vi "TSI Bench Single Socket CPV Sweeps E4990A Ver3.0.vi"() -> ()   [LabVIEW 2017]
uses:
  <vilib>/Utility/file.llb/Read Delimited Spreadsheet (DBL).vi
  Test Equipment/E364x/Agilent E364X Series/Agilent E364X Series.lvlib
  Test Equipment/KE2000/Keithley 2000/Keithley 2000.lvlib
panel:
  out "Cycles":string="2000"
  in  "Tab Control":enum32{"Control"}(tab)
  in  "Measure CMin \n& CMax Only?":bool
  in  "T- CAP(fF)":dbl[](array[numeric])=[100.0, 2968.75]
  out "Diff DCAP":dbl[](array[numeric])=[0.0, 158.76451612903202, 128.65967741935475, 83.51039999999999, 79.098, 80.17639999999999, 81.14560000000002, 79.77199999999999, 91.06439999999998, 80.7144, 80.3784, 79.76879999999998, 80.59799999999998, 91.3732, 90.2772]
  out "IDD ON (uA)":string
  out "I_Stdby (uA)":string
  out "CMax(fF)":dbl
  in  "Cycle?":bool=TRUE
  out "Cycles  No":i32=2000
  out "CMin (fF)":dbl=255.30700000000002
  in  "TP":string="TSI Bench Single Socket CPV Sweep E4990A Ver3.0"
  out "Error Out":errorcluster={"status"=FALSE, "code"=1073676407, "source"="VISA Open in Agilent E364X Series.lvlib:Initialize.vi->WS1021 Screen Parts Bench Test Ver1.4.vi"}
  in  "Base Path":path=path "C:/TSI Material"
  out "Status":string="Save Data..."
  in  "Tab Control 2":T1(tab)=enum."Input Info"
  in  "AGE364X":refnum<visa-resource-name>="GPIB0::6::INSTR"
  in  "VDD/VIO":dbl[](array[numeric])=[3.3, 1.8]
  in  "I_Limit (mA)":dbl=20.0 format="%.2p"
  in  "Select CPV":i32(ring)=17 items=["CP 24V", "CP 26V", "CP 28V", "CP 30V", "CP 31V", "CP 32V", "CP 33V", "CP 34V", "CP 35V", "CP 36V", "CP 37V", "CP 38V", "CP 39V", "CP 40V", "CP 41V", "CP 42V", "CP 43V", "CP 44V", "CP 45V", "CP 46V", "CP 47V", "CP 48V", "CP 49V", "CP 50V", "CP 51V", "CP 52V", "CP 53V", "CP 54V", "CP 56V", "CP 58V", "CP 60V", "CP 62V"]
  in  "Settings":bool
  in  "Comport Setting":refnum<visa-resource-name>="COM8"
  in  "Manual Write":string
  in  "Send":bool
  in  "No of Cycles":i32=2000
  in  "AG4990A":refnum<visa-resource-name>="GPIB0::17::INSTR"
  in  "KE2000":refnum<visa-resource-name>="GPIB0::9::INSTR"
  in  "Process Stop Button":bool
  in  "Stop":bool
  in  "Error In":errorcluster
  in  "CP CYC":bool
  in  "VDD":bool
  in  "Capacitance":bool
  in  "Info":T2={"Lot"="3127C", "Wafer"="11", "Package"="BC_C", "Device"="1"}
  out "IDD":cluster{dbl[], dbl[]}(graph)
  out "Cap Plot":cluster{dbl[], dbl[]}(graph)
  # "WiSpry Inc 20 Fairbanks \nSte 198 Irvine CA 92618\n\n\n\n\nRev Date = 07/27/2021\nTP:  TSI Bench Single Socket CPV Sweep E4990A Ver3.0\nLabVIEW 2017"
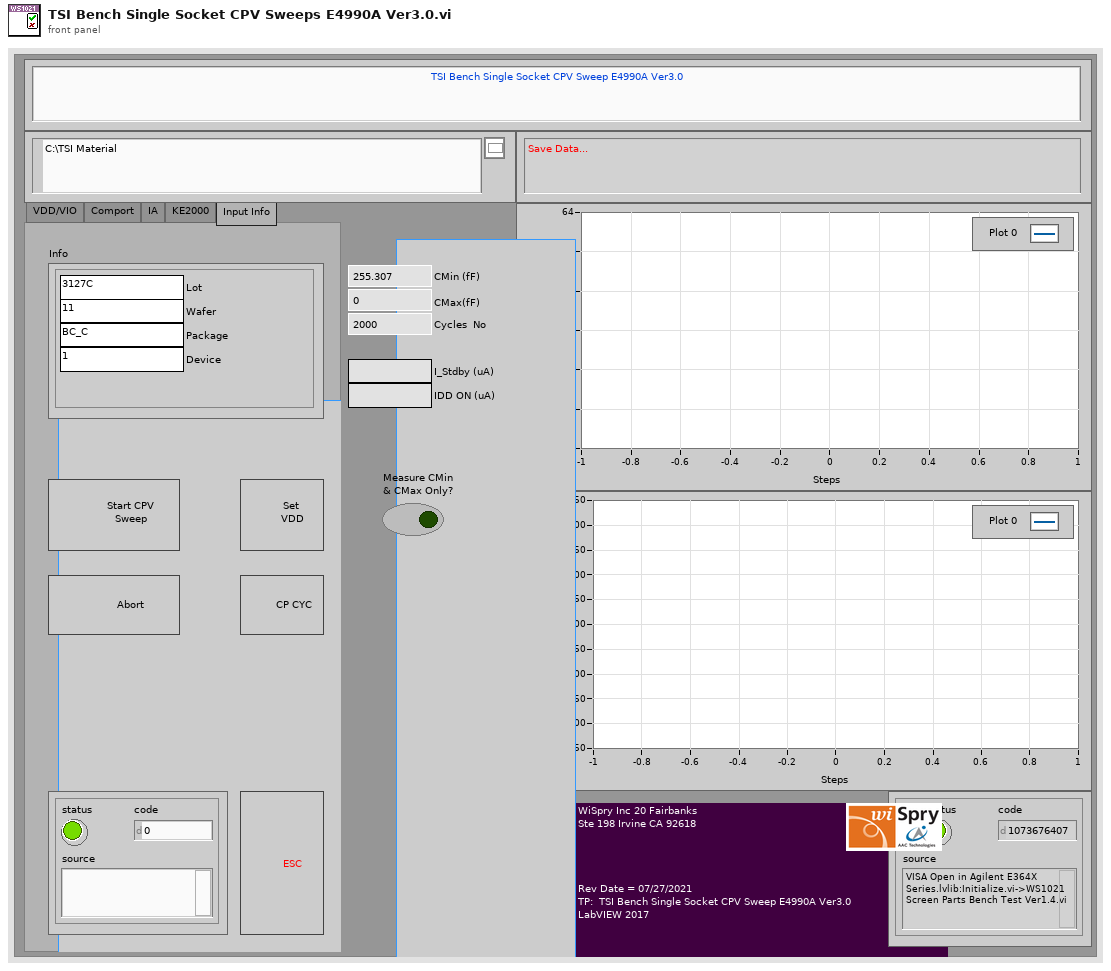
[diagram p1: front panel]
types:
  T1 = enum32{"VDD/VIO", "Comport", "IA", "KE2000", "Input Info"}
  T2 = cluster{"Lot":string, "Wafer":string, "Package":string, "Device":string}
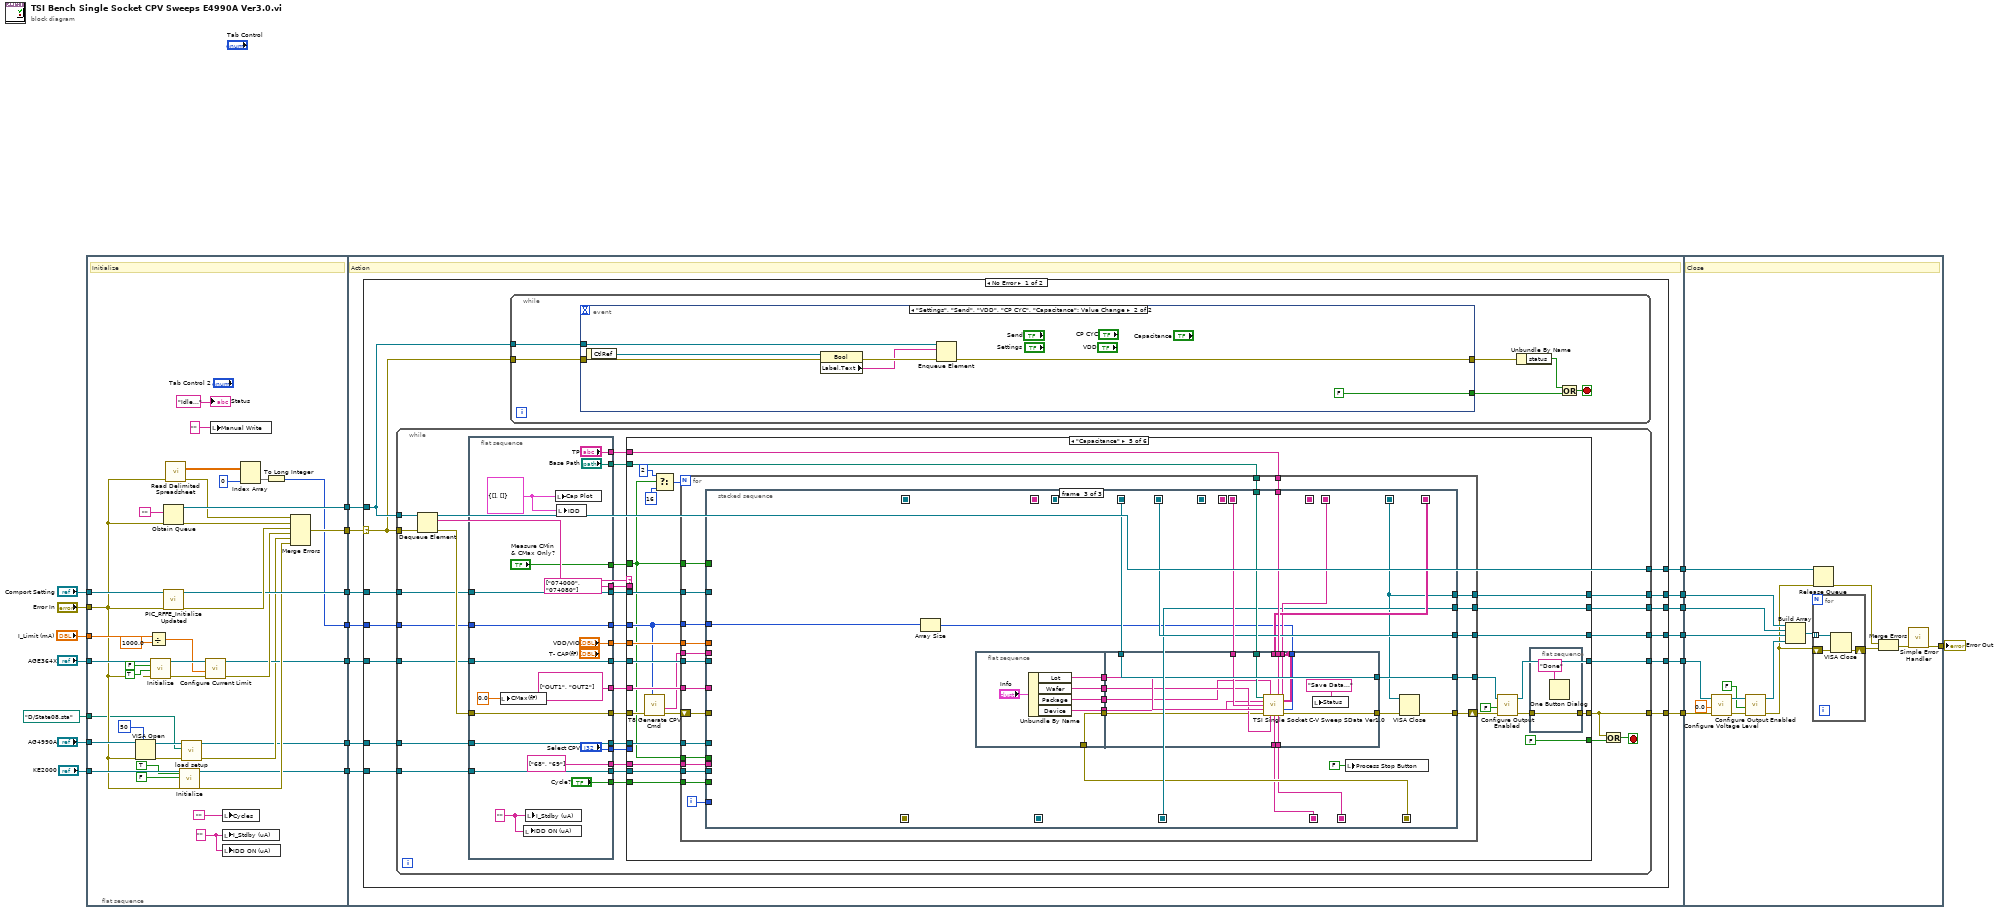
[diagram p0: block diagram]
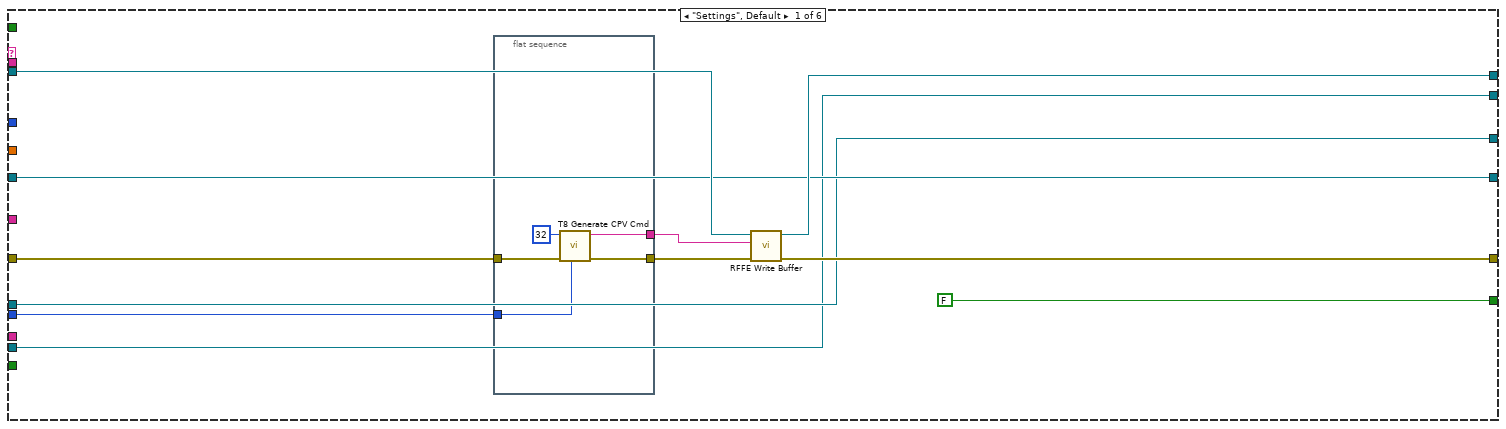
[diagram p2: hidden frame]
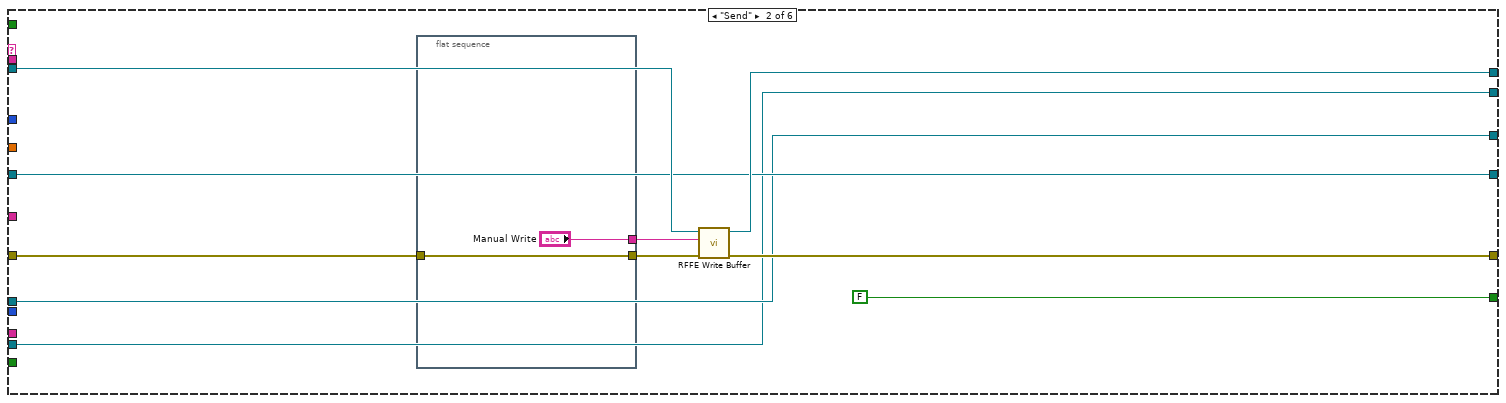
[diagram p3: hidden frame]
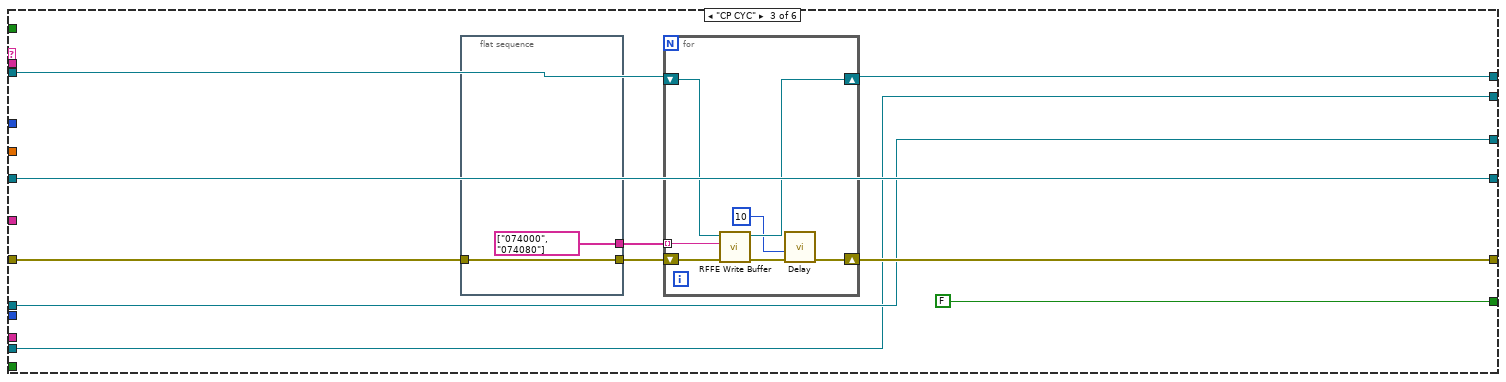
[diagram p4: hidden frame]
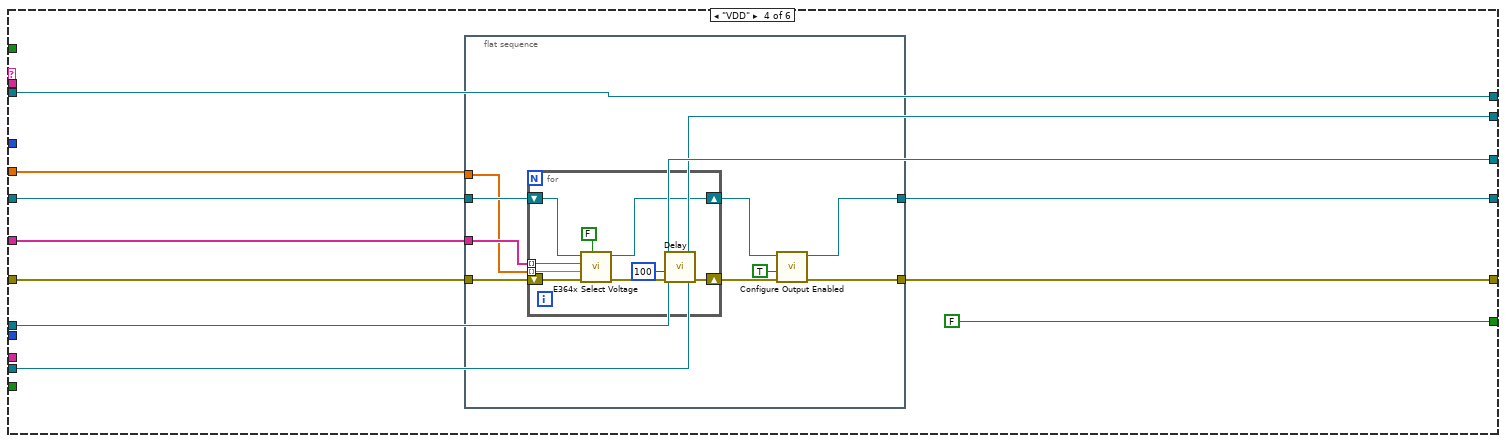
[diagram p5: hidden frame]
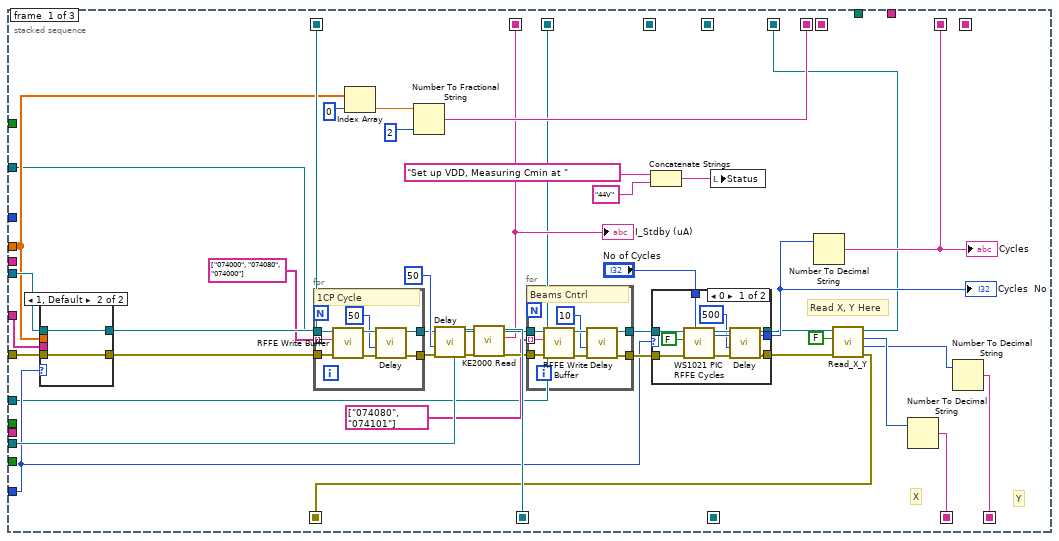
[diagram p6: hidden frame]
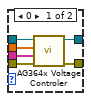
[diagram p7: hidden frame]
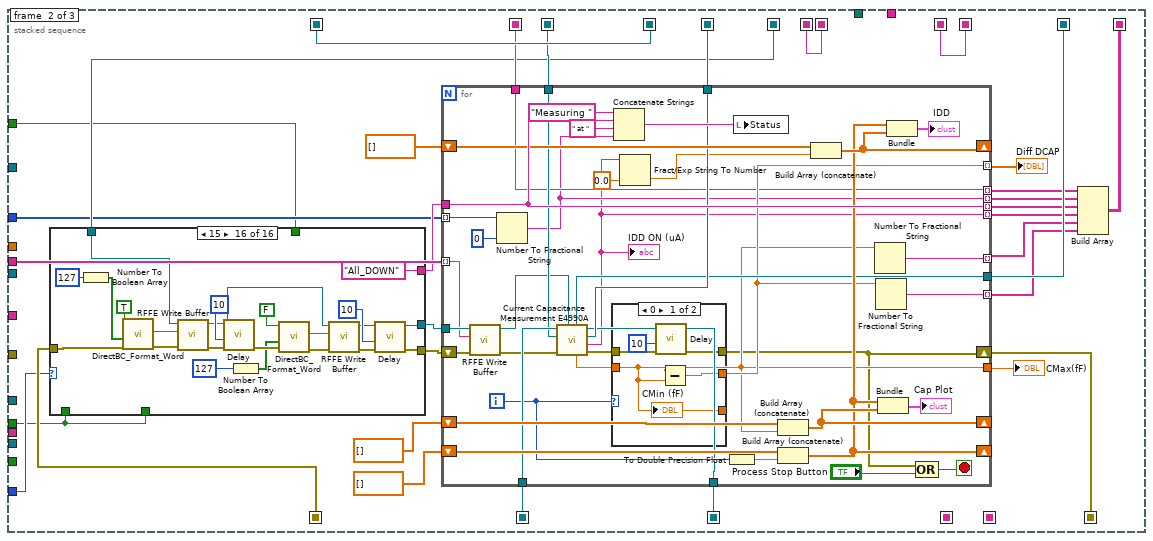
[diagram p9: hidden frame]
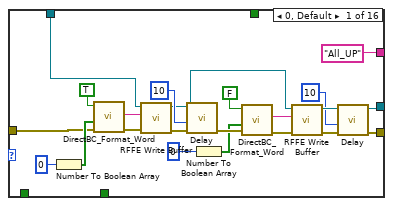
[diagram p10: hidden frame]
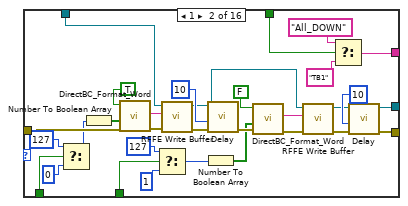
[diagram p11: hidden frame]
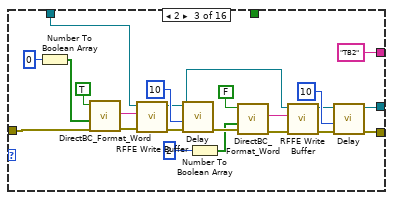
[diagram p12: hidden frame]
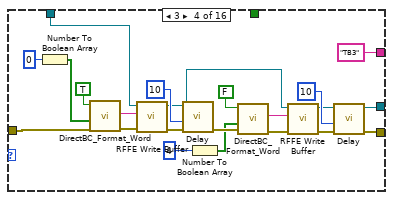
[diagram p13: hidden frame]
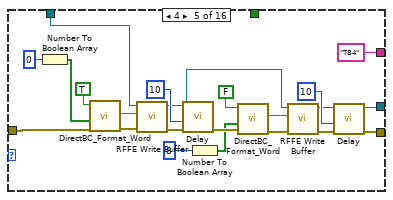
[diagram p14: hidden frame]
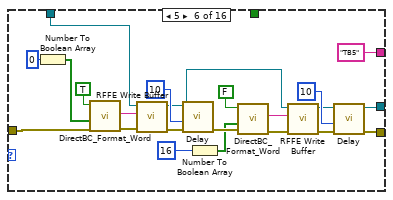
[diagram p15: hidden frame]
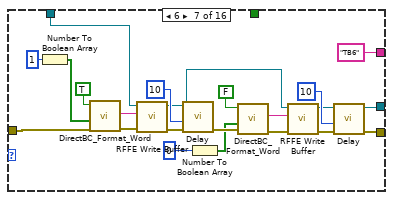
[diagram p16: hidden frame]
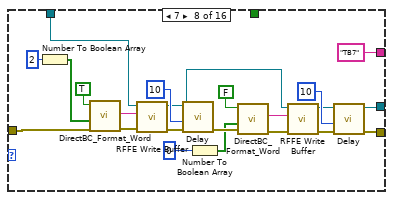
[diagram p17: hidden frame]
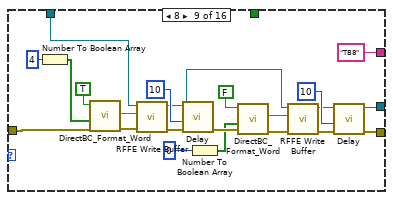
[diagram p18: hidden frame]
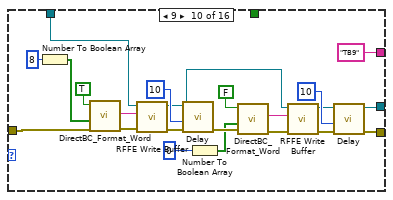
[diagram p19: hidden frame]
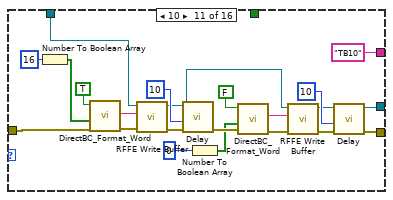
[diagram p20: hidden frame]
diagram:
  n1 = flat-sequence {
    tunnel: "Error In" -> [w28]
    tunnel: [w57] -> w20
    tunnel: [w59] -> w19
    tunnel: "Comport Setting" -> [w58]
    tunnel: [w54] -> w16
    tunnel: "AGE364X" -> [w52]
    tunnel: [w39] -> w12
    tunnel: "AG4990A" -> [w29]
    tunnel: [w24] -> w8
    tunnel: "KE2000" -> [w46]
    tunnel: [w43] -> w5
    tunnel: "I_Limit (mA)" -> [w38]
    tunnel: [w30] -> w2
    tunnel: path "D:/State08.sta" ("路径") -> [w23]
    tunnel: w20 -> [w69]
    tunnel: w19 -> [w73]
    tunnel: [w72] -> w18
    tunnel: w16 -> [w71]
    tunnel: [w70] -> w15
    tunnel: w12 -> [w68]
    tunnel: [w67] -> w11
    tunnel: [w66] -> w10
    tunnel: w8 -> [w65]
    tunnel: [w64] -> w7
    tunnel: w5 -> [w63]
    tunnel: [w62] -> w4
    tunnel: w2 -> [w61]
    tunnel: w18 -> [w862]
    tunnel: w15 -> [w848]
    tunnel: [w861] -> w14
    tunnel: w11 -> [w857]
    tunnel: w10 -> [w853]
    tunnel: w7 -> [w850]
    tunnel: w4 -> [w847]
    frame #0 {
      w35 = "" ("I_Stdby (uA)")
      # "Initialize"
      n2 = VISA Open(timeout (0)=u32 50 ("VISA Open timeout (0)"), error in (no error)=w28, VISA resource name=w29) -> (VISA resource name=w27:refnum<visa-resource-name>, error out=w26:errorcluster)  [unwired: 2 in]
      n3 = Divide(x=w38, y=1000.0) -> (x/y=w36:dbl)
      n4 = call "Initialize.vi"("error in (no error)"=w28, "ID Query (T: Query)"=TRUE, "Reset Device (T: Reset)"=FALSE, "VISA resource name"=w52) -> ("error out"=w41:errorcluster, "VISA resource name out"=w42:refnum<visa-resource-name>)  [unwired: 6 in]
      n5 = Obtain Queue(element data type="", error in (no error)=w28) -> (queue out=w59:refnum<queue>, error out=w56:errorcluster)  [unwired: 3 in, 1 out]
      n6 = call "PIC_RFFE_Initialize Updated.vi"("error in"=w28, "VISA In"=w58) -> ("error out"=w55:errorcluster, "VISA Out"=w54:refnum<visa-resource-name>)  [unwired: 8 in]
      n7 = call-poly <vilib>:"Read Delimited Spreadsheet.vi"("error in (no error)"=w28) -> ("all rows"=w34:dbl[][], "error out"=w31:errorcluster)  [unwired: 9 in, 4 out]
      n8 = call "Initialize.vi"("VISA resource name"=w46, "ID Query? (T: Check)"=TRUE, "Reset? (T: Reset)"=FALSE, "error in (no error)"=w28) -> ("VISA resource name out"=w43:refnum<visa-resource-name>, "error out"=w47:errorcluster)  [unwired: 14 in]
      n9 = call "load setup.vi"("错误输入（无错误）"=w26, "path"=w23, "VISA GPIB Resource"=w27) -> ("错误输出"=w25:errorcluster, "VISA资源名称输出"=w24:refnum<visa-resource-name>)  [unwired: 7 in]
      n10 = call "Configure Current Limit.vi"("error in (no error)"=w41, "Current Limit (0.0 Amps)"=w36, "VISA resource name"=w42) -> ("error out"=w40:errorcluster, "VISA resource name out"=w39:refnum<visa-resource-name>)  [unwired: 7 in]
      n11 = local write "Manual Write"("" ("Manual Write")) -> ()
      n12 = local write "Cycles"("") -> ()
      n13 = local write "I_Stdby (uA)"(w35) -> ()
      n14 = local write "IDD ON (uA)"(w35) -> ()
      n15 = Index Array(array=w34, index (col)=0 ("disabled index (col)")) -> (element=w32:dbl[])  [unwired: 1 in]
      n16 = To Long Integer(number=w32) -> (32bit integer=w30:i32[])
      n17 = Merge Errors(w31, w56, w55, w40, w25, w47) -> (w57:errorcluster)
      "Status" <- "Idle..." ("Status")
    }
    frame #1 {
      # "Action"
      n18 = case shown="No Error" w69 {
        selector: w69 -> [w82 w838]
        tunnel: w73 -> [w86 w840]
        tunnel: [w85 w840] -> w72
        tunnel: w71 -> [w84 w842]
        tunnel: [w83 w841] -> w70
        tunnel: w68 -> [w81 w839]
        tunnel: [w80 w837] -> w67
        tunnel: [w79 w839] -> w66
        tunnel: w65 -> [w78 w836]
        tunnel: [w77 w836] -> w64
        tunnel: w63 -> [w76 w835]
        tunnel: [w75 w835] -> w62
        tunnel: w61 -> [w74 _]
        frame No Error {
          n19 = while {
            tunnel: w86 -> [w118]
            tunnel: w82 -> [w117]
            tunnel: [w111] -> w85
            tunnel: w84 -> [w110]
            tunnel: [w108] -> w83
            tunnel: w81 -> [w107]
            tunnel: [w104] -> w79
            tunnel: [w99] -> w80
            tunnel: w78 -> [w102]
            tunnel: [w100] -> w77
            tunnel: w76 -> [w95]
            tunnel: [w93] -> w75
            tunnel: w74 -> [w89]
            stop <- w113 stop-if-true
            n20 = Dequeue Element(queue=w118, error in (no error)=w117) -> (queue out=w111:refnum<queue>, element=w116:string, error out=w115:errorcluster)  [unwired: 1 in, 1 out]
            n21 = flat-sequence {
              tunnel: w115 -> [w814]
              tunnel: [w814] -> w114
              tunnel: w110 -> [w813]
              tunnel: [w813] -> w109
              tunnel: w107 -> [w812]
              tunnel: [w812] -> w106
              tunnel: [string[] ["OUT1", "OUT2"]] -> w105
              tunnel: ["VDD/VIO"] -> w103
              tunnel: w102 -> [w810]
              tunnel: [w810] -> w101
              tunnel: ["Base Path"] -> w98
              tunnel: ["TP"] -> w97
              tunnel: ["Select CPV"] -> w96
              tunnel: w95 -> [w806]
              tunnel: [w806] -> w94
              tunnel: [string[] ["074000", "074080"]] -> w92
              tunnel: ["Cycle?"] -> w91
              tunnel: [string[] ["68", "69"]] -> w90
              tunnel: [w799] -> w88
              tunnel: w89 -> [w799]
              tunnel: ["Measure CMin \n& CMax Only?"] -> w87
              frame #0 {
                w801 = "" ("I_Stdby (uA)")
                w802 = cluster{dbl[], dbl[]} {[], []} ("Cap Plot")
                n22 = local write "CMax(fF)"(0.0 ("CMax(fF)")) -> ()
                n23 = local write "IDD ON (uA)"(w801) -> ()
                n24 = local write "I_Stdby (uA)"(w801) -> ()
                n25 = local write "Cap Plot"(w802) -> ()
                n26 = local write "IDD"(w802) -> ()
              }
            }
            n27 = case shown="\"Capacitance\"" w116 {
              tunnel: w114 -> [w129 w141 w153 w173 w201 w796]
              tunnel: [w126 w144 w156 w172 w204 w796] -> w99
              tunnel: [FALSE FALSE FALSE FALSE FALSE TRUE] -> w112
              tunnel: w109 -> [w125 w142 w154 w174 w215 w794]
              tunnel: [w124 w143 w155 w174 w214 w794] -> w108
              tunnel: w106 -> [w122 w137 w149 w171 w209 w793]
              tunnel: w105 -> [_ _ _ w170 w220 _]
              tunnel: [w122 w137 w149 w169 w203 w793] -> w104
              tunnel: w103 -> [_ _ _ w168 w221 _]
              tunnel: w101 -> [w121 w136 w148 w167 w211 w792]
              tunnel: [w121 w136 w148 w167 w210 w792] -> w100
              tunnel: w98 -> [_ _ _ _ w218 _]
              tunnel: w97 -> [_ _ _ _ w217 _]
              tunnel: w96 -> [w120 _ _ _ _ _]
              tunnel: w94 -> [w119 w135 w147 w166 w213 w791]
              tunnel: [w119 w135 w147 w166 w212 w791] -> w93
              tunnel: w92 -> [_ _ _ _ _ _]
              tunnel: w91 -> [_ _ _ _ w216 _]
              tunnel: w90 -> [_ _ _ _ w202 _]
              tunnel: w88 -> [_ _ _ _ w198 _]
              tunnel: w87 -> [_ _ _ _ w194 _]
              frame "Settings", Default {
                n28 = flat-sequence {
                  tunnel: w129 -> [w134]
                  tunnel: [w133] -> w127
                  tunnel: [w132] -> w123
                  tunnel: w120 -> [w130]
                  frame #0 {
                    n29 = call "T8 Generate CPV Cmd.vi"("Select CPV"=w130, "Error In"=w134, "Steps"=32) -> ("Error Out"=w133:errorcluster, "Cmd Send out"=w132:string)  [unwired: 5 in, 2 out]
                  }
                }
                n30 = call "RFFE Write Buffer.vi"("error in (no error)"=w127, "write buffer"=w123, "VISA resource name"=w125) -> ("error out"=w126:errorcluster, "VISA resource name out"=w124:refnum<visa-resource-name>)  [unwired: 7 in]
              }
              frame "Send" {
                n31 = flat-sequence {
                  tunnel: w141 -> [w146]
                  tunnel: [w146] -> w140
                  tunnel: ["Manual Write"] -> w139
                  frame #0 {
                  }
                }
                n32 = call "RFFE Write Buffer.vi"("error in (no error)"=w140, "write buffer"=w139, "VISA resource name"=w142) -> ("error out"=w144:errorcluster, "VISA resource name out"=w143:refnum<visa-resource-name>)  [unwired: 7 in]
              }
              frame "CP CYC" {
                n33 = flat-sequence {
                  tunnel: w153 -> [w165]
                  tunnel: [w165] -> w152
                  tunnel: [string[] ["074000", "074080"]] -> w151
                  frame #0 {
                  }
                }
                n34 = for {
                  tunnel: w151 -> [w160] mode=indexing
                  shift-right: [w163] -> w155
                  shift-left: w154 -> [w162]
                  shift-right: [w159] -> w156
                  shift-left: w152 -> [w161]
                  n35 = call "RFFE Write Buffer.vi"("error in (no error)"=w161, "write buffer"=w160, "VISA resource name"=w162) -> ("error out"=w158:errorcluster, "VISA resource name out"=w163:refnum<visa-resource-name>)  [unwired: 7 in]
                  n36 = call "Delay.vi"("error in (no error)"=w158, "Delay"=u32 10) -> ("error out"=w159:errorcluster)  [unwired: 9 in]
                }
              }
              frame "VDD" {
                n37 = flat-sequence {
                  tunnel: [w178] -> w169
                  tunnel: [w179] -> w172
                  tunnel: w171 -> [w183]
                  tunnel: w173 -> [w184]
                  tunnel: w170 -> [w182]
                  tunnel: w168 -> [w181]
                  frame #0 {
                    n38 = for {
                      shift-right: [w192] -> w180
                      shift-left: w184 -> [w193]
                      shift-right: [w185] -> w176
                      shift-left: w183 -> [w189]
                      tunnel: w182 -> [w188] mode=indexing
                      tunnel: w181 -> [w187] mode=indexing
                      n39 = call "E364x Select Voltage.vi"("Output Enabled (F: Off)"=FALSE, "error in"=w193, "Level (0.0 Volts)"=w187, "Output"=w188, "VISA in"=w189) -> ("error out"=w191:errorcluster, "VISA Out"=w185:refnum<visa-resource-name>)  [unwired: 5 in]
                      n40 = call "Delay.vi"("error in (no error)"=w191, "Delay"=u32 100) -> ("error out"=w192:errorcluster)  [unwired: 9 in]
                    }
                    n41 = call "Configure Output Enabled.vi"("error in (no error)"=w180, "Output Enabled (F: Off)"=TRUE, "VISA resource name"=w176) -> ("error out"=w179:errorcluster, "VISA resource name out"=w178:refnum<visa-resource-name>)  [unwired: 7 in]
                  }
                }
              }
              frame "Capacitance" {
                n42 = call "T8 Generate CPV Cmd.vi"("CP For Test"=w198, "Error In"=w201) -> ("Error Out"=w200:errorcluster, "Cmd Select"=w199:string[])  [unwired: 6 in, 2 out]
                n43 = Select(t=2, s=w194, f=16) -> (s? t:f=w196:i32)
                n44 = for {
                  N: w196 -> [_]
                  tunnel: w221 -> [w244]
                  tunnel: w220 -> [w243]
                  tunnel: w218 -> [w241]
                  tunnel: w217 -> [w239]
                  tunnel: w216 -> [w238]
                  shift-right: [w240] -> w207
                  shift-left: w200 -> [w242]
                  tunnel: w215 -> [w237]
                  tunnel: [w236] -> w214
                  tunnel: w213 -> [w235]
                  tunnel: [w234] -> w212
                  tunnel: w211 -> [w233]
                  tunnel: [w232] -> w210
                  tunnel: w209 -> [w231]
                  tunnel: [w230] -> w206
                  tunnel: w202 -> [w228]
                  tunnel: w199 -> [w227]
                  tunnel: w198 -> [w226]
                  tunnel: w194 -> [w225]
                  tunnel: w194 -> [w224]
                  i -> [w229]
                  n45 = stacked-sequence {
                    seq-local: [w248 _ _] -> [_ w330 _]
                    seq-local: [w281 _ _] -> [_ w348 _]
                    seq-local: [_ w350 _] -> [_ _ w759]
                    seq-local: [_ w349 _] -> [_ _ w752]
                    seq-local: [_ w348 _] -> [_ _ w768]
                    seq-local: [w276 _ _] -> [_ w347 _]
                    seq-local: [_ w347 _] -> [_ _ w764]
                    seq-local: [w255 _ _] -> [_ w346 _]
                    seq-local: [_ w345 _] -> [_ _ w763]
                    seq-local: [w249 _ _] -> [_ w329 _]
                    seq-local: [_ w343 _] -> [_ _ w762]
                    seq-local: [w270 _ _] -> [_ w342 _]
                    seq-local: [_ w342 _] -> [_ _ w761]
                    seq-local: [w265 _ _] -> [_ w336 _]
                    seq-local: [_ w335 _] -> [_ _ w760]
                    seq-local: [w259 _ _] -> [_ w332 _]
                    seq-local: [w253 _ _] -> [_ _ w746]
                    seq-local: [w252 _ _] -> [_ _ w747]
                    tunnel: w231 -> [w284 _ _]
                    tunnel: w244 -> [w277 _ _]
                    tunnel: w243 -> [w282 _ _]
                    tunnel: w242 -> [w283 _ _]
                    tunnel: w237 -> [w273 _ _]
                    tunnel: w233 -> [w255 _ _]
                    tunnel: [_ _ w767] -> w230
                    tunnel: w241 -> [_ _ w766]
                    tunnel: [_ _ w757] -> w240
                    tunnel: w239 -> [_ _ w765]
                    tunnel: [_ _ w763] -> w232
                    tunnel: [_ _ w759] -> w236
                    tunnel: w235 -> [w266 _ _]
                    tunnel: [_ _ w760] -> w234
                    tunnel: w238 -> [_ _ _]
                    tunnel: w229 -> [w256 w326 _]
                    tunnel: w228 -> [_ _ _]
                    tunnel: w227 -> [_ w327 _]
                    tunnel: w226 -> [_ w322 w749]
                    tunnel: w225 -> [_ w320 _]
                    tunnel: w224 -> [_ w319 _]
                    frame #0 {
                      # "Y"
                      # "X"
                      # "Read X, Y Here"
                      n46 = case shown="1, Default" w256 {
                        tunnel: w284 -> [w290 w291]
                        tunnel: w283 -> [w289 w292]
                        tunnel: w282 -> [w288 _]
                        tunnel: [w287 w291] -> w281
                        tunnel: w277 -> [w286 _]
                        tunnel: [w285 w292] -> w274
                        frame 0 {
                          n47 = call "AG364x Voltage Controler.vi"("error in (no error)"=w289, "Select CH"=w288, "VDD/VIO"=w286, "VISA In"=w290) -> ("error out"=w285:errorcluster, "VISA Out"=w287:refnum<visa-resource-name>)  [unwired: 6 in]
                        }
                        frame 1, Default {
                        }
                      }
                      n48 = for {
                        tunnel: [w314] -> w268
                        tunnel: string[] ["074000", "074080", "074000"] -> [w318] mode=indexing
                        tunnel: w274 -> [w317]
                        tunnel: w273 -> [w316]
                        tunnel: [w315] -> w261
                        # "1CP Cycle"
                        n49 = call "RFFE Write Buffer.vi"("error in (no error)"=w317, "write buffer"=w318, "VISA resource name"=w316) -> ("error out"=w313:errorcluster, "VISA resource name out"=w315:refnum<visa-resource-name>)  [unwired: 7 in]
                        n50 = call "Delay.vi"("error in (no error)"=w313, "Delay"=u32 50) -> ("error out"=w314:errorcluster)  [unwired: 9 in]
                      }
                      n51 = Index Array(array=w277, index=0) -> (element=w280:dbl)
                      n52 = Number To Fractional String(number=w280, precision (6)=i16 2) -> (F-format string=w276:string)  [unwired: 2 in]
                      n53 = call "Delay.vi"("error in (no error)"=w268, "Delay"=u32 50) -> ("error out"=w269:errorcluster)  [unwired: 9 in]
                      n54 = call "KE2000 Read.vi"("error in (no error)"=w269, "VISA resource name"=w266) -> ("error out"=w263:errorcluster, "uA"=w259:string, "VISA resource name out"=w265:refnum<visa-resource-name>)  [unwired: 7 in]
                      "I_Stdby (uA)" <- w259
                      n55 = for {
                        tunnel: [w295] -> w264
                        tunnel: string[] ["074080", "074101"] -> [w299] mode=indexing
                        tunnel: w263 -> [w298]
                        tunnel: w261 -> [w297]
                        tunnel: [w296] -> w260
                        # "Beams Cntrl"
                        n56 = call "RFFE Write Buffer.vi"("error in (no error)"=w298, "write buffer"=w299, "VISA resource name"=w297) -> ("error out"=w294:errorcluster, "VISA resource name out"=w296:refnum<visa-resource-name>)  [unwired: 7 in]
                        n57 = call "Delay.vi"("error in (no error)"=w294, "Delay"=u32 10) -> ("error out"=w295:errorcluster)  [unwired: 9 in]
                      }
                      n58 = Concatenate Strings("Set up VDD, Measuring Cmin at " ("Status"), "44V" ("string")) -> (w257:string)
                      n59 = case shown="0" w256 {
                        tunnel: w260 -> [w307 w311]
                        tunnel: w264 -> [w306 w309]
                        tunnel: [w301 w309] -> w251
                        tunnel: [w305 w311] -> w250
                        tunnel: [w304 w310] -> w271
                        tunnel: "No of Cycles" -> [w303 w310]
                        frame 0 {
                          n60 = call "WS1021 PIC RFFE Cycles.vi"("No of Cycles"=w303, "Error In"=w306, "Init"=FALSE, "VISA In"=w307) -> ("Error Out"=w302:errorcluster, "VISA Out"=w305:refnum<visa-resource-name>, "Cycles Completed"=w304:i32)  [unwired: 5 in]
                          n61 = call "Delay.vi"("error in (no error)"=w302, "Delay"=u32 500) -> ("error out"=w301:errorcluster)  [unwired: 9 in]
                        }
                        frame 1, Default {
                        }
                      }
                      "Cycles  No" <- w271
                      n62 = local write "Status"(w257) -> ()
                      n63 = Number To Decimal String(number=w271) -> (decimal integer string=w270:string)  [unwired: 1 in]
                      "Cycles" <- w270
                      n64 = call "Read_X_Y.vi"("error in (no error)"=w251, "PIC Init?"=FALSE, "VISA resource name"=w250) -> ("error out"=w248:errorcluster, "Y"=w245:u32, "X"=w246:u32, "VISA resource name out"=w249:refnum<visa-resource-name>)  [unwired: 5 in]
                      n65 = Number To Decimal String(number=w246) -> (decimal integer string=w252:string)  [unwired: 1 in]
                      n66 = Number To Decimal String(number=w245) -> (decimal integer string=w253:string)  [unwired: 1 in]
                    }
                    frame #1 {
                      n67 = case shown="15" w326 {
                        tunnel: w330 -> [w352 w385 w403 w424 w445 w466 w487 w508 w529 w550 w571 w592 w613 w634 w655 w676]
                        tunnel: w329 -> [w351 w386 w404 w425 w446 w467 w488 w509 w530 w551 w572 w593 w614 w635 w656 w677]
                        tunnel: [w370 w387 w405 w426 w447 w468 w489 w510 w531 w552 w573 w594 w615 w636 w657 w678] -> w328
                        tunnel: [w371 w384 w402 w423 w444 w465 w486 w507 w528 w549 w570 w591 w612 w633 w654 w675] -> w325
                        tunnel: ["All_UP" w373 "TB2" "TB3" "TB4" "TB5" "TB6" "TB7" "TB8" "TB9" "TB10" "TB11" "FB1" "FB2" "FB3" "All_DOWN"] -> w324
                        tunnel: w320 -> [_ w378 _ _ _ _ _ _ _ _ _ _ _ _ _ _]
                        tunnel: w320 -> [_ w377 _ _ _ _ _ _ _ _ _ _ _ _ _ _]
                        tunnel: w319 -> [_ w375 _ _ _ _ _ _ _ _ _ _ _ _ _ _]
                        frame 0, Default {
                          n68 = Number To Boolean Array(number=0) -> (Boolean array=w363:bool[])
                          n69 = call "DirectBC_Format_Word.vi"("error in (no error)"=w352, "DC Reg Settings"=w363, "Reg2?\nTrue/False = Reg2/ Reg 3"=TRUE ("Reg2?\nTrue/False = Reg2/ Reg 3")) -> ("error out"=w361:errorcluster, "Direct Beam Control Word Out"=w360:string)  [unwired: 7 in]
                          n70 = call "RFFE Write Buffer.vi"("error in (no error)"=w361, "write buffer"=w360, "VISA resource name"=w351) -> ("error out"=w365:errorcluster, "VISA resource name out"=w354:refnum<visa-resource-name>)  [unwired: 7 in]
                          n71 = call "Delay.vi"("error in (no error)"=w365, "Delay"=u32 10) -> ("error out"=w359:errorcluster)  [unwired: 9 in]
                          n72 = Number To Boolean Array(number=0) -> (Boolean array=w357:bool[])
                          n73 = call "DirectBC_Format_Word.vi"("error in (no error)"=w359, "DC Reg Settings"=w357, "Reg2?\nTrue/False = Reg2/ Reg 3"=FALSE ("Reg2?\nTrue/False = Reg2/ Reg 3")) -> ("error out"=w355:errorcluster, "Direct Beam Control Word Out"=w353:string)  [unwired: 7 in]
                          n74 = call "RFFE Write Buffer.vi"("error in (no error)"=w355, "write buffer"=w353, "VISA resource name"=w354) -> ("error out"=w368:errorcluster, "VISA resource name out"=w370:refnum<visa-resource-name>)  [unwired: 7 in]
                          n75 = call "Delay.vi"("error in (no error)"=w368, "Delay"=u32 10) -> ("error out"=w371:errorcluster)  [unwired: 9 in]
                        }
                        frame 1 {
                          n76 = Select(t=127 ("number"), s=w378, f=0 ("number")) -> (s? t:f=w380:i32)
                          n77 = Number To Boolean Array(number=w380) -> (Boolean array=w396:bool[])
                          n78 = call "DirectBC_Format_Word.vi"("error in (no error)"=w385, "DC Reg Settings"=w396, "Reg2?\nTrue/False = Reg2/ Reg 3"=TRUE ("Reg2?\nTrue/False = Reg2/ Reg 3")) -> ("error out"=w395:errorcluster, "Direct Beam Control Word Out"=w394:string)  [unwired: 7 in]
                          n79 = Select(t=127 ("number"), s=w377, f=1 ("number")) -> (s? t:f=w383:i32)
                          n80 = call "RFFE Write Buffer.vi"("error in (no error)"=w395, "write buffer"=w394, "VISA resource name"=w386) -> ("error out"=w398:errorcluster, "VISA resource name out"=w389:refnum<visa-resource-name>)  [unwired: 7 in]
                          n81 = Number To Boolean Array(number=w383) -> (Boolean array=w391:bool[])
                          n82 = call "Delay.vi"("error in (no error)"=w398, "Delay"=u32 10) -> ("error out"=w393:errorcluster)  [unwired: 9 in]
                          n83 = call "DirectBC_Format_Word.vi"("error in (no error)"=w393, "DC Reg Settings"=w391, "Reg2?\nTrue/False = Reg2/ Reg 3"=FALSE ("Reg2?\nTrue/False = Reg2/ Reg 3")) -> ("error out"=w390:errorcluster, "Direct Beam Control Word Out"=w388:string)  [unwired: 7 in]
                          n84 = call "RFFE Write Buffer.vi"("error in (no error)"=w390, "write buffer"=w388, "VISA resource name"=w389) -> ("error out"=w401:errorcluster, "VISA resource name out"=w387:refnum<visa-resource-name>)  [unwired: 7 in]
                          n85 = Select(t="All_DOWN", s=w375, f="TB1") -> (s? t:f=w373:string)
                          n86 = call "Delay.vi"("error in (no error)"=w401, "Delay"=u32 10) -> ("error out"=w384:errorcluster)  [unwired: 9 in]
                        }
                        frame 2 {
                          n87 = Number To Boolean Array(number=0) -> (Boolean array=w416:bool[])
                          n88 = call "DirectBC_Format_Word.vi"("error in (no error)"=w403, "DC Reg Settings"=w416, "Reg2?\nTrue/False = Reg2/ Reg 3"=TRUE ("Reg2?\nTrue/False = Reg2/ Reg 3")) -> ("error out"=w414:errorcluster, "Direct Beam Control Word Out"=w413:string)  [unwired: 7 in]
                          n89 = call "RFFE Write Buffer.vi"("error in (no error)"=w414, "write buffer"=w413, "VISA resource name"=w404) -> ("error out"=w418:errorcluster, "VISA resource name out"=w407:refnum<visa-resource-name>)  [unwired: 7 in]
                          n90 = call "Delay.vi"("error in (no error)"=w418, "Delay"=u32 10) -> ("error out"=w412:errorcluster)  [unwired: 9 in]
                          n91 = Number To Boolean Array(number=2) -> (Boolean array=w410:bool[])
                          n92 = call "DirectBC_Format_Word.vi"("error in (no error)"=w412, "DC Reg Settings"=w410, "Reg2?\nTrue/False = Reg2/ Reg 3"=FALSE ("Reg2?\nTrue/False = Reg2/ Reg 3")) -> ("error out"=w408:errorcluster, "Direct Beam Control Word Out"=w406:string)  [unwired: 7 in]
                          n93 = call "RFFE Write Buffer.vi"("error in (no error)"=w408, "write buffer"=w406, "VISA resource name"=w407) -> ("error out"=w421:errorcluster, "VISA resource name out"=w405:refnum<visa-resource-name>)  [unwired: 7 in]
                          n94 = call "Delay.vi"("error in (no error)"=w421, "Delay"=u32 10) -> ("error out"=w402:errorcluster)  [unwired: 9 in]
                        }
                        frame 3 {
                          n95 = Number To Boolean Array(number=0) -> (Boolean array=w437:bool[])
                          n96 = call "DirectBC_Format_Word.vi"("error in (no error)"=w424, "DC Reg Settings"=w437, "Reg2?\nTrue/False = Reg2/ Reg 3"=TRUE ("Reg2?\nTrue/False = Reg2/ Reg 3")) -> ("error out"=w435:errorcluster, "Direct Beam Control Word Out"=w434:string)  [unwired: 7 in]
                          n97 = call "RFFE Write Buffer.vi"("error in (no error)"=w435, "write buffer"=w434, "VISA resource name"=w425) -> ("error out"=w439:errorcluster, "VISA resource name out"=w428:refnum<visa-resource-name>)  [unwired: 7 in]
                          n98 = call "Delay.vi"("error in (no error)"=w439, "Delay"=u32 10) -> ("error out"=w433:errorcluster)  [unwired: 9 in]
                          n99 = Number To Boolean Array(number=4) -> (Boolean array=w431:bool[])
                          n100 = call "DirectBC_Format_Word.vi"("error in (no error)"=w433, "DC Reg Settings"=w431, "Reg2?\nTrue/False = Reg2/ Reg 3"=FALSE ("Reg2?\nTrue/False = Reg2/ Reg 3")) -> ("error out"=w429:errorcluster, "Direct Beam Control Word Out"=w427:string)  [unwired: 7 in]
                          n101 = call "RFFE Write Buffer.vi"("error in (no error)"=w429, "write buffer"=w427, "VISA resource name"=w428) -> ("error out"=w442:errorcluster, "VISA resource name out"=w426:refnum<visa-resource-name>)  [unwired: 7 in]
                          n102 = call "Delay.vi"("error in (no error)"=w442, "Delay"=u32 10) -> ("error out"=w423:errorcluster)  [unwired: 9 in]
                        }
                        frame 4 {
                          n103 = Number To Boolean Array(number=0) -> (Boolean array=w458:bool[])
                          n104 = call "DirectBC_Format_Word.vi"("error in (no error)"=w445, "DC Reg Settings"=w458, "Reg2?\nTrue/False = Reg2/ Reg 3"=TRUE ("Reg2?\nTrue/False = Reg2/ Reg 3")) -> ("error out"=w456:errorcluster, "Direct Beam Control Word Out"=w455:string)  [unwired: 7 in]
                          n105 = call "RFFE Write Buffer.vi"("error in (no error)"=w456, "write buffer"=w455, "VISA resource name"=w446) -> ("error out"=w460:errorcluster, "VISA resource name out"=w449:refnum<visa-resource-name>)  [unwired: 7 in]
                          n106 = call "Delay.vi"("error in (no error)"=w460, "Delay"=u32 10) -> ("error out"=w454:errorcluster)  [unwired: 9 in]
                          n107 = Number To Boolean Array(number=8) -> (Boolean array=w452:bool[])
                          n108 = call "DirectBC_Format_Word.vi"("error in (no error)"=w454, "DC Reg Settings"=w452, "Reg2?\nTrue/False = Reg2/ Reg 3"=FALSE ("Reg2?\nTrue/False = Reg2/ Reg 3")) -> ("error out"=w450:errorcluster, "Direct Beam Control Word Out"=w448:string)  [unwired: 7 in]
                          n109 = call "RFFE Write Buffer.vi"("error in (no error)"=w450, "write buffer"=w448, "VISA resource name"=w449) -> ("error out"=w463:errorcluster, "VISA resource name out"=w447:refnum<visa-resource-name>)  [unwired: 7 in]
                          n110 = call "Delay.vi"("error in (no error)"=w463, "Delay"=u32 10) -> ("error out"=w444:errorcluster)  [unwired: 9 in]
                        }
                        frame 5 {
                          n111 = Number To Boolean Array(number=0) -> (Boolean array=w479:bool[])
                          n112 = call "DirectBC_Format_Word.vi"("error in (no error)"=w466, "DC Reg Settings"=w479, "Reg2?\nTrue/False = Reg2/ Reg 3"=TRUE ("Reg2?\nTrue/False = Reg2/ Reg 3")) -> ("error out"=w477:errorcluster, "Direct Beam Control Word Out"=w476:string)  [unwired: 7 in]
                          n113 = call "RFFE Write Buffer.vi"("error in (no error)"=w477, "write buffer"=w476, "VISA resource name"=w467) -> ("error out"=w481:errorcluster, "VISA resource name out"=w470:refnum<visa-resource-name>)  [unwired: 7 in]
                          n114 = call "Delay.vi"("error in (no error)"=w481, "Delay"=u32 10) -> ("error out"=w475:errorcluster)  [unwired: 9 in]
                          n115 = Number To Boolean Array(number=16) -> (Boolean array=w473:bool[])
                          n116 = call "DirectBC_Format_Word.vi"("error in (no error)"=w475, "DC Reg Settings"=w473, "Reg2?\nTrue/False = Reg2/ Reg 3"=FALSE ("Reg2?\nTrue/False = Reg2/ Reg 3")) -> ("error out"=w471:errorcluster, "Direct Beam Control Word Out"=w469:string)  [unwired: 7 in]
                          n117 = call "RFFE Write Buffer.vi"("error in (no error)"=w471, "write buffer"=w469, "VISA resource name"=w470) -> ("error out"=w484:errorcluster, "VISA resource name out"=w468:refnum<visa-resource-name>)  [unwired: 7 in]
                          n118 = call "Delay.vi"("error in (no error)"=w484, "Delay"=u32 10) -> ("error out"=w465:errorcluster)  [unwired: 9 in]
                        }
                        frame 6 {
                          n119 = Number To Boolean Array(number=1) -> (Boolean array=w500:bool[])
                          n120 = call "DirectBC_Format_Word.vi"("error in (no error)"=w487, "DC Reg Settings"=w500, "Reg2?\nTrue/False = Reg2/ Reg 3"=TRUE ("Reg2?\nTrue/False = Reg2/ Reg 3")) -> ("error out"=w498:errorcluster, "Direct Beam Control Word Out"=w497:string)  [unwired: 7 in]
                          n121 = call "RFFE Write Buffer.vi"("error in (no error)"=w498, "write buffer"=w497, "VISA resource name"=w488) -> ("error out"=w502:errorcluster, "VISA resource name out"=w491:refnum<visa-resource-name>)  [unwired: 7 in]
                          n122 = call "Delay.vi"("error in (no error)"=w502, "Delay"=u32 10) -> ("error out"=w496:errorcluster)  [unwired: 9 in]
                          n123 = Number To Boolean Array(number=0) -> (Boolean array=w494:bool[])
                          n124 = call "DirectBC_Format_Word.vi"("error in (no error)"=w496, "DC Reg Settings"=w494, "Reg2?\nTrue/False = Reg2/ Reg 3"=FALSE ("Reg2?\nTrue/False = Reg2/ Reg 3")) -> ("error out"=w492:errorcluster, "Direct Beam Control Word Out"=w490:string)  [unwired: 7 in]
                          n125 = call "RFFE Write Buffer.vi"("error in (no error)"=w492, "write buffer"=w490, "VISA resource name"=w491) -> ("error out"=w505:errorcluster, "VISA resource name out"=w489:refnum<visa-resource-name>)  [unwired: 7 in]
                          n126 = call "Delay.vi"("error in (no error)"=w505, "Delay"=u32 10) -> ("error out"=w486:errorcluster)  [unwired: 9 in]
                        }
                        frame 7 {
                          n127 = Number To Boolean Array(number=2) -> (Boolean array=w521:bool[])
                          n128 = call "DirectBC_Format_Word.vi"("error in (no error)"=w508, "DC Reg Settings"=w521, "Reg2?\nTrue/False = Reg2/ Reg 3"=TRUE ("Reg2?\nTrue/False = Reg2/ Reg 3")) -> ("error out"=w519:errorcluster, "Direct Beam Control Word Out"=w518:string)  [unwired: 7 in]
                          n129 = call "RFFE Write Buffer.vi"("error in (no error)"=w519, "write buffer"=w518, "VISA resource name"=w509) -> ("error out"=w523:errorcluster, "VISA resource name out"=w512:refnum<visa-resource-name>)  [unwired: 7 in]
                          n130 = call "Delay.vi"("error in (no error)"=w523, "Delay"=u32 10) -> ("error out"=w517:errorcluster)  [unwired: 9 in]
                          n131 = Number To Boolean Array(number=0) -> (Boolean array=w515:bool[])
                          n132 = call "DirectBC_Format_Word.vi"("error in (no error)"=w517, "DC Reg Settings"=w515, "Reg2?\nTrue/False = Reg2/ Reg 3"=FALSE ("Reg2?\nTrue/False = Reg2/ Reg 3")) -> ("error out"=w513:errorcluster, "Direct Beam Control Word Out"=w511:string)  [unwired: 7 in]
                          n133 = call "RFFE Write Buffer.vi"("error in (no error)"=w513, "write buffer"=w511, "VISA resource name"=w512) -> ("error out"=w526:errorcluster, "VISA resource name out"=w510:refnum<visa-resource-name>)  [unwired: 7 in]
                          n134 = call "Delay.vi"("error in (no error)"=w526, "Delay"=u32 10) -> ("error out"=w507:errorcluster)  [unwired: 9 in]
                        }
                        frame 8 {
                          n135 = Number To Boolean Array(number=4) -> (Boolean array=w542:bool[])
                          n136 = call "DirectBC_Format_Word.vi"("error in (no error)"=w529, "DC Reg Settings"=w542, "Reg2?\nTrue/False = Reg2/ Reg 3"=TRUE ("Reg2?\nTrue/False = Reg2/ Reg 3")) -> ("error out"=w540:errorcluster, "Direct Beam Control Word Out"=w539:string)  [unwired: 7 in]
                          n137 = call "RFFE Write Buffer.vi"("error in (no error)"=w540, "write buffer"=w539, "VISA resource name"=w530) -> ("error out"=w544:errorcluster, "VISA resource name out"=w533:refnum<visa-resource-name>)  [unwired: 7 in]
                          n138 = call "Delay.vi"("error in (no error)"=w544, "Delay"=u32 10) -> ("error out"=w538:errorcluster)  [unwired: 9 in]
                          n139 = Number To Boolean Array(number=0) -> (Boolean array=w536:bool[])
                          n140 = call "DirectBC_Format_Word.vi"("error in (no error)"=w538, "DC Reg Settings"=w536, "Reg2?\nTrue/False = Reg2/ Reg 3"=FALSE ("Reg2?\nTrue/False = Reg2/ Reg 3")) -> ("error out"=w534:errorcluster, "Direct Beam Control Word Out"=w532:string)  [unwired: 7 in]
                          n141 = call "RFFE Write Buffer.vi"("error in (no error)"=w534, "write buffer"=w532, "VISA resource name"=w533) -> ("error out"=w547:errorcluster, "VISA resource name out"=w531:refnum<visa-resource-name>)  [unwired: 7 in]
                          n142 = call "Delay.vi"("error in (no error)"=w547, "Delay"=u32 10) -> ("error out"=w528:errorcluster)  [unwired: 9 in]
                        }
                        frame 9 {
                          n143 = Number To Boolean Array(number=8) -> (Boolean array=w563:bool[])
                          n144 = call "DirectBC_Format_Word.vi"("error in (no error)"=w550, "DC Reg Settings"=w563, "Reg2?\nTrue/False = Reg2/ Reg 3"=TRUE ("Reg2?\nTrue/False = Reg2/ Reg 3")) -> ("error out"=w561:errorcluster, "Direct Beam Control Word Out"=w560:string)  [unwired: 7 in]
                          n145 = call "RFFE Write Buffer.vi"("error in (no error)"=w561, "write buffer"=w560, "VISA resource name"=w551) -> ("error out"=w565:errorcluster, "VISA resource name out"=w554:refnum<visa-resource-name>)  [unwired: 7 in]
                          n146 = call "Delay.vi"("error in (no error)"=w565, "Delay"=u32 10) -> ("error out"=w559:errorcluster)  [unwired: 9 in]
                          n147 = Number To Boolean Array(number=0) -> (Boolean array=w557:bool[])
                          n148 = call "DirectBC_Format_Word.vi"("error in (no error)"=w559, "DC Reg Settings"=w557, "Reg2?\nTrue/False = Reg2/ Reg 3"=FALSE ("Reg2?\nTrue/False = Reg2/ Reg 3")) -> ("error out"=w555:errorcluster, "Direct Beam Control Word Out"=w553:string)  [unwired: 7 in]
                          n149 = call "RFFE Write Buffer.vi"("error in (no error)"=w555, "write buffer"=w553, "VISA resource name"=w554) -> ("error out"=w568:errorcluster, "VISA resource name out"=w552:refnum<visa-resource-name>)  [unwired: 7 in]
                          n150 = call "Delay.vi"("error in (no error)"=w568, "Delay"=u32 10) -> ("error out"=w549:errorcluster)  [unwired: 9 in]
                        }
                        frame 10 {
                          n151 = Number To Boolean Array(number=16) -> (Boolean array=w584:bool[])
                          n152 = call "DirectBC_Format_Word.vi"("error in (no error)"=w571, "DC Reg Settings"=w584, "Reg2?\nTrue/False = Reg2/ Reg 3"=TRUE ("Reg2?\nTrue/False = Reg2/ Reg 3")) -> ("error out"=w582:errorcluster, "Direct Beam Control Word Out"=w581:string)  [unwired: 7 in]
                          n153 = call "RFFE Write Buffer.vi"("error in (no error)"=w582, "write buffer"=w581, "VISA resource name"=w572) -> ("error out"=w586:errorcluster, "VISA resource name out"=w575:refnum<visa-resource-name>)  [unwired: 7 in]
                          n154 = call "Delay.vi"("error in (no error)"=w586, "Delay"=u32 10) -> ("error out"=w580:errorcluster)  [unwired: 9 in]
                          n155 = Number To Boolean Array(number=0) -> (Boolean array=w578:bool[])
                          n156 = call "DirectBC_Format_Word.vi"("error in (no error)"=w580, "DC Reg Settings"=w578, "Reg2?\nTrue/False = Reg2/ Reg 3"=FALSE ("Reg2?\nTrue/False = Reg2/ Reg 3")) -> ("error out"=w576:errorcluster, "Direct Beam Control Word Out"=w574:string)  [unwired: 7 in]
                          n157 = call "RFFE Write Buffer.vi"("error in (no error)"=w576, "write buffer"=w574, "VISA resource name"=w575) -> ("error out"=w589:errorcluster, "VISA resource name out"=w573:refnum<visa-resource-name>)  [unwired: 7 in]
                          n158 = call "Delay.vi"("error in (no error)"=w589, "Delay"=u32 10) -> ("error out"=w570:errorcluster)  [unwired: 9 in]
                        }
                        frame 11 {
                          n159 = Number To Boolean Array(number=32) -> (Boolean array=w605:bool[])
                          n160 = call "DirectBC_Format_Word.vi"("error in (no error)"=w592, "DC Reg Settings"=w605, "Reg2?\nTrue/False = Reg2/ Reg 3"=TRUE ("Reg2?\nTrue/False = Reg2/ Reg 3")) -> ("error out"=w603:errorcluster, "Direct Beam Control Word Out"=w602:string)  [unwired: 7 in]
                          n161 = call "RFFE Write Buffer.vi"("error in (no error)"=w603, "write buffer"=w602, "VISA resource name"=w593) -> ("error out"=w607:errorcluster, "VISA resource name out"=w596:refnum<visa-resource-name>)  [unwired: 7 in]
                          n162 = call "Delay.vi"("error in (no error)"=w607, "Delay"=u32 10) -> ("error out"=w601:errorcluster)  [unwired: 9 in]
                          n163 = Number To Boolean Array(number=0) -> (Boolean array=w599:bool[])
                          n164 = call "DirectBC_Format_Word.vi"("error in (no error)"=w601, "DC Reg Settings"=w599, "Reg2?\nTrue/False = Reg2/ Reg 3"=FALSE ("Reg2?\nTrue/False = Reg2/ Reg 3")) -> ("error out"=w597:errorcluster, "Direct Beam Control Word Out"=w595:string)  [unwired: 7 in]
                          n165 = call "RFFE Write Buffer.vi"("error in (no error)"=w597, "write buffer"=w595, "VISA resource name"=w596) -> ("error out"=w610:errorcluster, "VISA resource name out"=w594:refnum<visa-resource-name>)  [unwired: 7 in]
                          n166 = call "Delay.vi"("error in (no error)"=w610, "Delay"=u32 10) -> ("error out"=w591:errorcluster)  [unwired: 9 in]
                        }
                        frame 12 {
                          n167 = Number To Boolean Array(number=0) -> (Boolean array=w626:bool[])
                          n168 = call "DirectBC_Format_Word.vi"("error in (no error)"=w613, "DC Reg Settings"=w626, "Reg2?\nTrue/False = Reg2/ Reg 3"=TRUE ("Reg2?\nTrue/False = Reg2/ Reg 3")) -> ("error out"=w624:errorcluster, "Direct Beam Control Word Out"=w623:string)  [unwired: 7 in]
                          n169 = call "RFFE Write Buffer.vi"("error in (no error)"=w624, "write buffer"=w623, "VISA resource name"=w614) -> ("error out"=w628:errorcluster, "VISA resource name out"=w617:refnum<visa-resource-name>)  [unwired: 7 in]
                          n170 = call "Delay.vi"("error in (no error)"=w628, "Delay"=u32 10) -> ("error out"=w622:errorcluster)  [unwired: 9 in]
                          n171 = Number To Boolean Array(number=64) -> (Boolean array=w620:bool[])
                          n172 = call "DirectBC_Format_Word.vi"("error in (no error)"=w622, "DC Reg Settings"=w620, "Reg2?\nTrue/False = Reg2/ Reg 3"=FALSE ("Reg2?\nTrue/False = Reg2/ Reg 3")) -> ("error out"=w618:errorcluster, "Direct Beam Control Word Out"=w616:string)  [unwired: 7 in]
                          n173 = call "RFFE Write Buffer.vi"("error in (no error)"=w618, "write buffer"=w616, "VISA resource name"=w617) -> ("error out"=w631:errorcluster, "VISA resource name out"=w615:refnum<visa-resource-name>)  [unwired: 7 in]
                          n174 = call "Delay.vi"("error in (no error)"=w631, "Delay"=u32 10) -> ("error out"=w612:errorcluster)  [unwired: 9 in]
                        }
                        frame 13 {
                          n175 = Number To Boolean Array(number=64) -> (Boolean array=w647:bool[])
                          n176 = call "DirectBC_Format_Word.vi"("error in (no error)"=w634, "DC Reg Settings"=w647, "Reg2?\nTrue/False = Reg2/ Reg 3"=TRUE ("Reg2?\nTrue/False = Reg2/ Reg 3")) -> ("error out"=w645:errorcluster, "Direct Beam Control Word Out"=w644:string)  [unwired: 7 in]
                          n177 = call "RFFE Write Buffer.vi"("error in (no error)"=w645, "write buffer"=w644, "VISA resource name"=w635) -> ("error out"=w649:errorcluster, "VISA resource name out"=w638:refnum<visa-resource-name>)  [unwired: 7 in]
                          n178 = call "Delay.vi"("error in (no error)"=w649, "Delay"=u32 10) -> ("error out"=w643:errorcluster)  [unwired: 9 in]
                          n179 = Number To Boolean Array(number=0) -> (Boolean array=w641:bool[])
                          n180 = call "DirectBC_Format_Word.vi"("error in (no error)"=w643, "DC Reg Settings"=w641, "Reg2?\nTrue/False = Reg2/ Reg 3"=FALSE ("Reg2?\nTrue/False = Reg2/ Reg 3")) -> ("error out"=w639:errorcluster, "Direct Beam Control Word Out"=w637:string)  [unwired: 7 in]
                          n181 = call "RFFE Write Buffer.vi"("error in (no error)"=w639, "write buffer"=w637, "VISA resource name"=w638) -> ("error out"=w652:errorcluster, "VISA resource name out"=w636:refnum<visa-resource-name>)  [unwired: 7 in]
                          n182 = call "Delay.vi"("error in (no error)"=w652, "Delay"=u32 10) -> ("error out"=w633:errorcluster)  [unwired: 9 in]
                        }
                        frame 14 {
                          n183 = Number To Boolean Array(number=0) -> (Boolean array=w668:bool[])
                          n184 = call "DirectBC_Format_Word.vi"("error in (no error)"=w655, "DC Reg Settings"=w668, "Reg2?\nTrue/False = Reg2/ Reg 3"=TRUE ("Reg2?\nTrue/False = Reg2/ Reg 3")) -> ("error out"=w666:errorcluster, "Direct Beam Control Word Out"=w665:string)  [unwired: 7 in]
                          n185 = call "RFFE Write Buffer.vi"("error in (no error)"=w666, "write buffer"=w665, "VISA resource name"=w656) -> ("error out"=w670:errorcluster, "VISA resource name out"=w659:refnum<visa-resource-name>)  [unwired: 7 in]
                          n186 = call "Delay.vi"("error in (no error)"=w670, "Delay"=u32 10) -> ("error out"=w664:errorcluster)  [unwired: 9 in]
                          n187 = Number To Boolean Array(number=32) -> (Boolean array=w662:bool[])
                          n188 = call "DirectBC_Format_Word.vi"("error in (no error)"=w664, "DC Reg Settings"=w662, "Reg2?\nTrue/False = Reg2/ Reg 3"=FALSE ("Reg2?\nTrue/False = Reg2/ Reg 3")) -> ("error out"=w660:errorcluster, "Direct Beam Control Word Out"=w658:string)  [unwired: 7 in]
                          n189 = call "RFFE Write Buffer.vi"("error in (no error)"=w660, "write buffer"=w658, "VISA resource name"=w659) -> ("error out"=w673:errorcluster, "VISA resource name out"=w657:refnum<visa-resource-name>)  [unwired: 7 in]
                          n190 = call "Delay.vi"("error in (no error)"=w673, "Delay"=u32 10) -> ("error out"=w654:errorcluster)  [unwired: 9 in]
                        }
                        frame 15 {
                          n191 = Number To Boolean Array(number=127) -> (Boolean array=w689:bool[])
                          n192 = call "DirectBC_Format_Word.vi"("error in (no error)"=w676, "DC Reg Settings"=w689, "Reg2?\nTrue/False = Reg2/ Reg 3"=TRUE ("Reg2?\nTrue/False = Reg2/ Reg 3")) -> ("error out"=w687:errorcluster, "Direct Beam Control Word Out"=w686:string)  [unwired: 7 in]
                          n193 = call "RFFE Write Buffer.vi"("error in (no error)"=w687, "write buffer"=w686, "VISA resource name"=w677) -> ("error out"=w691:errorcluster, "VISA resource name out"=w680:refnum<visa-resource-name>)  [unwired: 7 in]
                          n194 = call "Delay.vi"("error in (no error)"=w691, "Delay"=u32 10) -> ("error out"=w685:errorcluster)  [unwired: 9 in]
                          n195 = Number To Boolean Array(number=127) -> (Boolean array=w683:bool[])
                          n196 = call "DirectBC_Format_Word.vi"("error in (no error)"=w685, "DC Reg Settings"=w683, "Reg2?\nTrue/False = Reg2/ Reg 3"=FALSE ("Reg2?\nTrue/False = Reg2/ Reg 3")) -> ("error out"=w681:errorcluster, "Direct Beam Control Word Out"=w679:string)  [unwired: 7 in]
                          n197 = call "RFFE Write Buffer.vi"("error in (no error)"=w681, "write buffer"=w679, "VISA resource name"=w680) -> ("error out"=w694:errorcluster, "VISA resource name out"=w678:refnum<visa-resource-name>)  [unwired: 7 in]
                          n198 = call "Delay.vi"("error in (no error)"=w694, "Delay"=u32 10) -> ("error out"=w675:errorcluster)  [unwired: 9 in]
                        }
                      }
                      n199 = for {
                        shift-right: [w696] -> w349
                        shift-left: w325 -> [w713]
                        tunnel: [w707] -> w350
                        tunnel: [w708] -> w345
                        tunnel: w346 -> [w720]
                        tunnel: w324 -> [w733]
                        tunnel: [w729] -> w344 mode=indexing
                        tunnel: [w733] -> w333 mode=indexing
                        tunnel: [w701] -> w341 mode=indexing
                        tunnel: [w705] -> w340 mode=indexing
                        tunnel: [w699] -> w334 mode=indexing
                        shift-right: [w724] -> _
                        shift-left: dbl[] [] -> [w731]
                        shift-right: [w726] -> _
                        shift-left: dbl[] [] -> [w730]
                        shift-right: [w723] -> _
                        shift-left: dbl[] [] -> [w728]
                        tunnel: w336 -> [w721]
                        tunnel: [w706] -> w335
                        tunnel: [w718] -> w323 mode=indexing
                        tunnel: w332 -> [w704]
                        tunnel: [w704] -> w331 mode=indexing
                        tunnel: [w700] -> w321
                        tunnel: w328 -> [w710]
                        tunnel: w327 -> [w709] mode=indexing
                        tunnel: w322 -> [w702] mode=indexing
                        i -> [w714]
                        stop <- w715 stop-if-true
                        n200 = call "RFFE Write Buffer.vi"("error in (no error)"=w713, "write buffer"=w709, "VISA resource name"=w710) -> ("error out"=w712:errorcluster, "VISA resource name out"=w711:refnum<visa-resource-name>)  [unwired: 7 in]
                        n201 = Number To Fractional String(number=w702, precision (6)=i16 0) -> (F-format string=w701:string)  [unwired: 2 in]
                        n202 = call "Current Capacitance Measurement E4990A.vi"("RFFE In"=w711, "Error In"=w712, "E4980A LCR In"=w720, "KE2000 In"=w721) -> ("Error Out"=w719:errorcluster, "uA"=w699:string, "E4980A LCR Out"=w708:refnum<visa-resource-name>, "KE2000 Out"=w706:refnum<visa-resource-name>, "Cap(fF)"=w700:dbl, "RFFE Out"=w707:refnum<visa-resource-name>)  [unwired: 2 in]
                        "IDD ON (uA)" <- w699
                        n203 = case shown="0" w714 {
                          tunnel: [w739 w745] -> w696
                          tunnel: w719 -> [w738 w744]
                          tunnel: w700 -> [w736 w740]
                          tunnel: [w736 w741] -> _
                          tunnel: [w735 w742] -> w705
                          frame 0 {
                            n204 = call "Delay.vi"("error in (no error)"=w738, "Delay"=u32 10) -> ("error out"=w739:errorcluster)  [unwired: 9 in]
                            n205 = Subtract(x=w736, y=w736) -> (x-y=w735:dbl)
                            "CMin (fF)" <- w736
                          }
                          frame 1, Default {
                            n206 = local read "CMin (fF)"() -> (w741:dbl)
                            n207 = call "Delay.vi"("error in (no error)"=w744, "Delay"=u32 10) -> ("error out"=w745:errorcluster)  [unwired: 9 in]
                            n208 = Subtract(x=w740, y=w741) -> (x-y=w742:dbl)
                          }
                        }
                        n209 = Concatenate Strings("Measuring " ("Status"), w733, " at " ("string"), w701) -> (w732:string)
                        n210 = Fract/Exp String To Number(string=w699, default (0 dbl)=0.0 ("default (0 DBL)")) -> (number=w698:dbl)  [unwired: 2 in, 1 out]
                        n211 = To Double Precision Float(number=w714) -> (double precision float=w727:dbl)
                        n212 = local write "Status"(w732) -> ()
                        n213 = Build Array (concatenate)(w730, w700) -> (w726:dbl[])
                        n214 = Build Array (concatenate)(w728, w727) -> (w723:dbl[])
                        n215 = Build Array (concatenate)(w731, w698) -> (w724:dbl[])
                        n216 = Number To Fractional String(number=w700) -> (F-format string=w729:string)  [unwired: 3 in]
                        n217 = Number To Fractional String(number=w705) -> (F-format string=w718:string)  [unwired: 3 in]
                        n218 = Bundle(w723, w726) -> (→"Cap Plot":cluster{dbl[], dbl[]})  [unwired: 1 in]
                        n219 = Bundle(w723, w724) -> (→"IDD":cluster{dbl[], dbl[]})  [unwired: 1 in]
                        n220 = Compound Arithmetic op=OR(w696, "Process Stop Button") -> (w715:bool)
                      }
                      "Diff DCAP" <- w340
                      "CMax(fF)" <- w321
                      n221 = Build Array(w331, w341, w333, w334, w344, w323) -> (w343:string[][])
                    }
                    frame #2 {
                      n222 = Array Size(array=w749) -> (size(s)=w748:i32)
                      n223 = flat-sequence {
                        tunnel: [w773] -> w756
                        tunnel: [w772] -> w755
                        tunnel: [w771] -> w754
                        tunnel: [w770] -> w753
                        tunnel: w752 -> [w769]
                        tunnel: [w769] -> w751
                        tunnel: [w790] -> w767
                        tunnel: [w789] -> w758
                        tunnel: w768 -> [w790]
                        tunnel: w761 -> [w783]
                        tunnel: w762 -> [w785]
                        tunnel: [w785] -> _
                        tunnel: w764 -> [w786]
                        tunnel: w765 -> [w787]
                        tunnel: w766 -> [w788]
                        tunnel: w756 -> [w782]
                        tunnel: w755 -> [w781]
                        tunnel: w754 -> [w780]
                        tunnel: w753 -> [w779]
                        tunnel: w751 -> [w778]
                        tunnel: w748 -> [w777]
                        tunnel: w747 -> [w776]
                        tunnel: w746 -> [w775]
                        frame #0 {
                          n224 = Unbundle By Name("Info") -> ("Lot"=w773:string, "Wafer"=w772:string, "Package"=w770:string, "Device"=w771:string)
                        }
                        frame #1 {
                          n225 = call "TSI Single Socket C-V Sweep SData Ver1.0.vi"("Base Path"=w788, "Package"=w779, "Data In"=w785, "TP"=w787, "Cyc"=w783, "Cell"=w780, "VDD To PGR OTP"=w786, "Lot"=w782, "Index"=w777, "error in (no error)"=w778, "Wafer"=w781, "X"=w776, "Y"=w775) -> ("error out"=w789:errorcluster)  [unwired: 2 in]
                          n226 = local write "Status"("Save Data..." ("Status")) -> ()
                        }
                      }
                      n227 = local write "Process Stop Button"(FALSE ("Process Stop Button")) -> ()
                      n228 = VISA Close(VISA resource name=w759, error in (no error)=w758) -> (error out=w757:errorcluster)
                    }
                  }
                }
                n229 = call "Configure Output Enabled.vi"("error in (no error)"=w207, "Output Enabled (F: Off)"=FALSE, "VISA resource name"=w206) -> ("error out"=w205:errorcluster, "VISA resource name out"=w203:refnum<visa-resource-name>)  [unwired: 7 in]
                n230 = flat-sequence {
                  tunnel: w205 -> [w222]
                  tunnel: [w222] -> w204
                  frame #0 {
                    n231 = One Button Dialog(message="Done") -> ()  [unwired: 1 in, 1 out]
                  }
                }
              }
              frame "Stop" {
              }
            }
            n232 = Or(x=w99, y=w112) -> (x .or. y?=w113:bool)
          }
          n233 = while {
            tunnel: w82 -> [w820]
            tunnel: w86 -> [w819]
            stop <- w818 stop-if-true
            n234 = event shown="[1] \"Settings\", \"Send\", \"VDD\", \"CP CYC\", \"Capacitance\": Value Change" {
              selector: _ -> [_ _]
              dyn-events: _ -> [_ _]
              timeout: _ -> [_ _]
              tunnel: [TRUE ("Stop") FALSE ("Stop")] -> w816
              tunnel: w820 -> [w825 w832]
              tunnel: w819 -> [w827 w834]
              tunnel: [w822 w829] -> w815
              event "Stop": Value Change {
                n235 = event-data() -> ("CtlRef"=w826:refnum<vi>)  [unwired: 1 in]
                n236 = property class="Bool"(reference=w826, error in=w825) -> (error out=w824:errorcluster, "Label.Text"=w823:string)  [unwired: 1 out]
                n237 = Enqueue Element(queue=w827, element=w823, error in (no error)=w824) -> (error out=w822:errorcluster)  [unwired: 1 in, 2 out]
              }
              event "Settings", "Send", "VDD", "CP CYC", "Capacitance": Value Change {
                n238 = event-data() -> ("CtlRef"=w833:refnum<vi>)  [unwired: 1 in]
                n239 = property class="Bool"(reference=w833, error in=w832) -> (error out=w831:errorcluster, "Label.Text"=w830:string)  [unwired: 1 out]
                n240 = Enqueue Element(queue=w834, element=w830, error in (no error)=w831) -> (error out=w829:errorcluster)  [unwired: 1 in, 2 out]
              }
            }
            n241 = Unbundle By Name(w815) -> ("status"=w817:bool)
            n242 = Or(x=w817, y=w816) -> (x .or. y?=w818:bool)
          }
        }
        frame Error {
          n243 = flat-sequence {
            tunnel: [w844] -> w841
            tunnel: w842 -> [w844]
            tunnel: [w843] -> w837
            tunnel: w838 -> [w843]
            frame #0 {
              n244 = One Button Dialog(message="Check Comport") -> ()  [unwired: 1 in, 1 out]
            }
          }
        }
      }
    }
    frame #2 {
      # "Close"
      n245 = call "Configure Voltage Level.vi"("error in (no error)"=w857, "Level (0.0 Volts)"=0.0, "VISA resource name"=w853) -> ("error out"=w856:errorcluster, "VISA resource name out"=w860:refnum<visa-resource-name>)  [unwired: 7 in]
      n246 = call "Configure Output Enabled.vi"("error in (no error)"=w856, "Output Enabled (F: Off)"=FALSE, "VISA resource name"=w860) -> ("error out"=w846:errorcluster, "VISA resource name out"=w849:refnum<visa-resource-name>)  [unwired: 7 in]
      n247 = Build Array(w848, w847, w850, w849) -> (w851:refnum<visa-resource-name>[])
      n248 = for {
        tunnel: w851 -> [w865] mode=indexing
        shift-right: [w864] -> w852
        shift-left: w846 -> [w863]
        n249 = VISA Close(VISA resource name=w865, error in (no error)=w863) -> (error out=w864:errorcluster)
      }
      n250 = Release Queue(queue=w862, error in (no error)=w846) -> (error out=w855:errorcluster)  [unwired: 1 in, 2 out]
      n251 = Merge Errors(w855, w852) -> (w854:errorcluster)
      n252 = call <vilib>:"Simple Error Handler.vi"("error in (no error)"=w854) -> ("error out"=w861:errorcluster)  [unwired: 4 in, 4 out]
    }
  }
  "Error Out" <- w14
